vi "FE FF Frame Decoder.vi"(4 "Limit Enable(T)":bool=TRUE, 5 "INFO":T1, 6 "Test Mode":u32, 7 "Raw_Data?":bool=TRUE, 8 "error in (no error)":errorcluster, 10 "Frame Data":u8[](array[numeric]), 11 "Frame Detail":string[][](array[string])) -> (0 "error out":errorcluster, 2 "Raw Data":u64[](array[numeric]), 3 "Frame Detail With Value":string[](array[string]))   [LabVIEW 2023, in "HardwareAbstractionLayer_LVOOP.lvlib" / "Report.lvclass"]
uses:
  Report.lvclass
  Control/FE FF DECODER.ctl
  Control/ERROR LOG.ctl
  Control/TEST RESULT LOG.ctl
  Control/All Log Details.ctl
  Control/UUT Test Info.ctl
  Control/FE FRAME LOG.ctl
  Control/FF FRAME LOG.ctl
  Control/LIMIT TABLE.ctl
  Control/ERROR LOG APPEND.ctl
  Control/FA FRAME LOG.ctl
  Control/TEST RESULT LOG APPEND.ctl
  Control/SYSTEM LOG.ctl
  Control/Temperature LOG.ctl
  Control/POWER STATUS.ctl
  Control/CYCLE_DURATION_LOG.ctl
  <vilib>/Utility/error.llb/Trim Whitespace One-Sided.vi
  Report.lvclass/Report.ctl
  Database/Database.lvclass
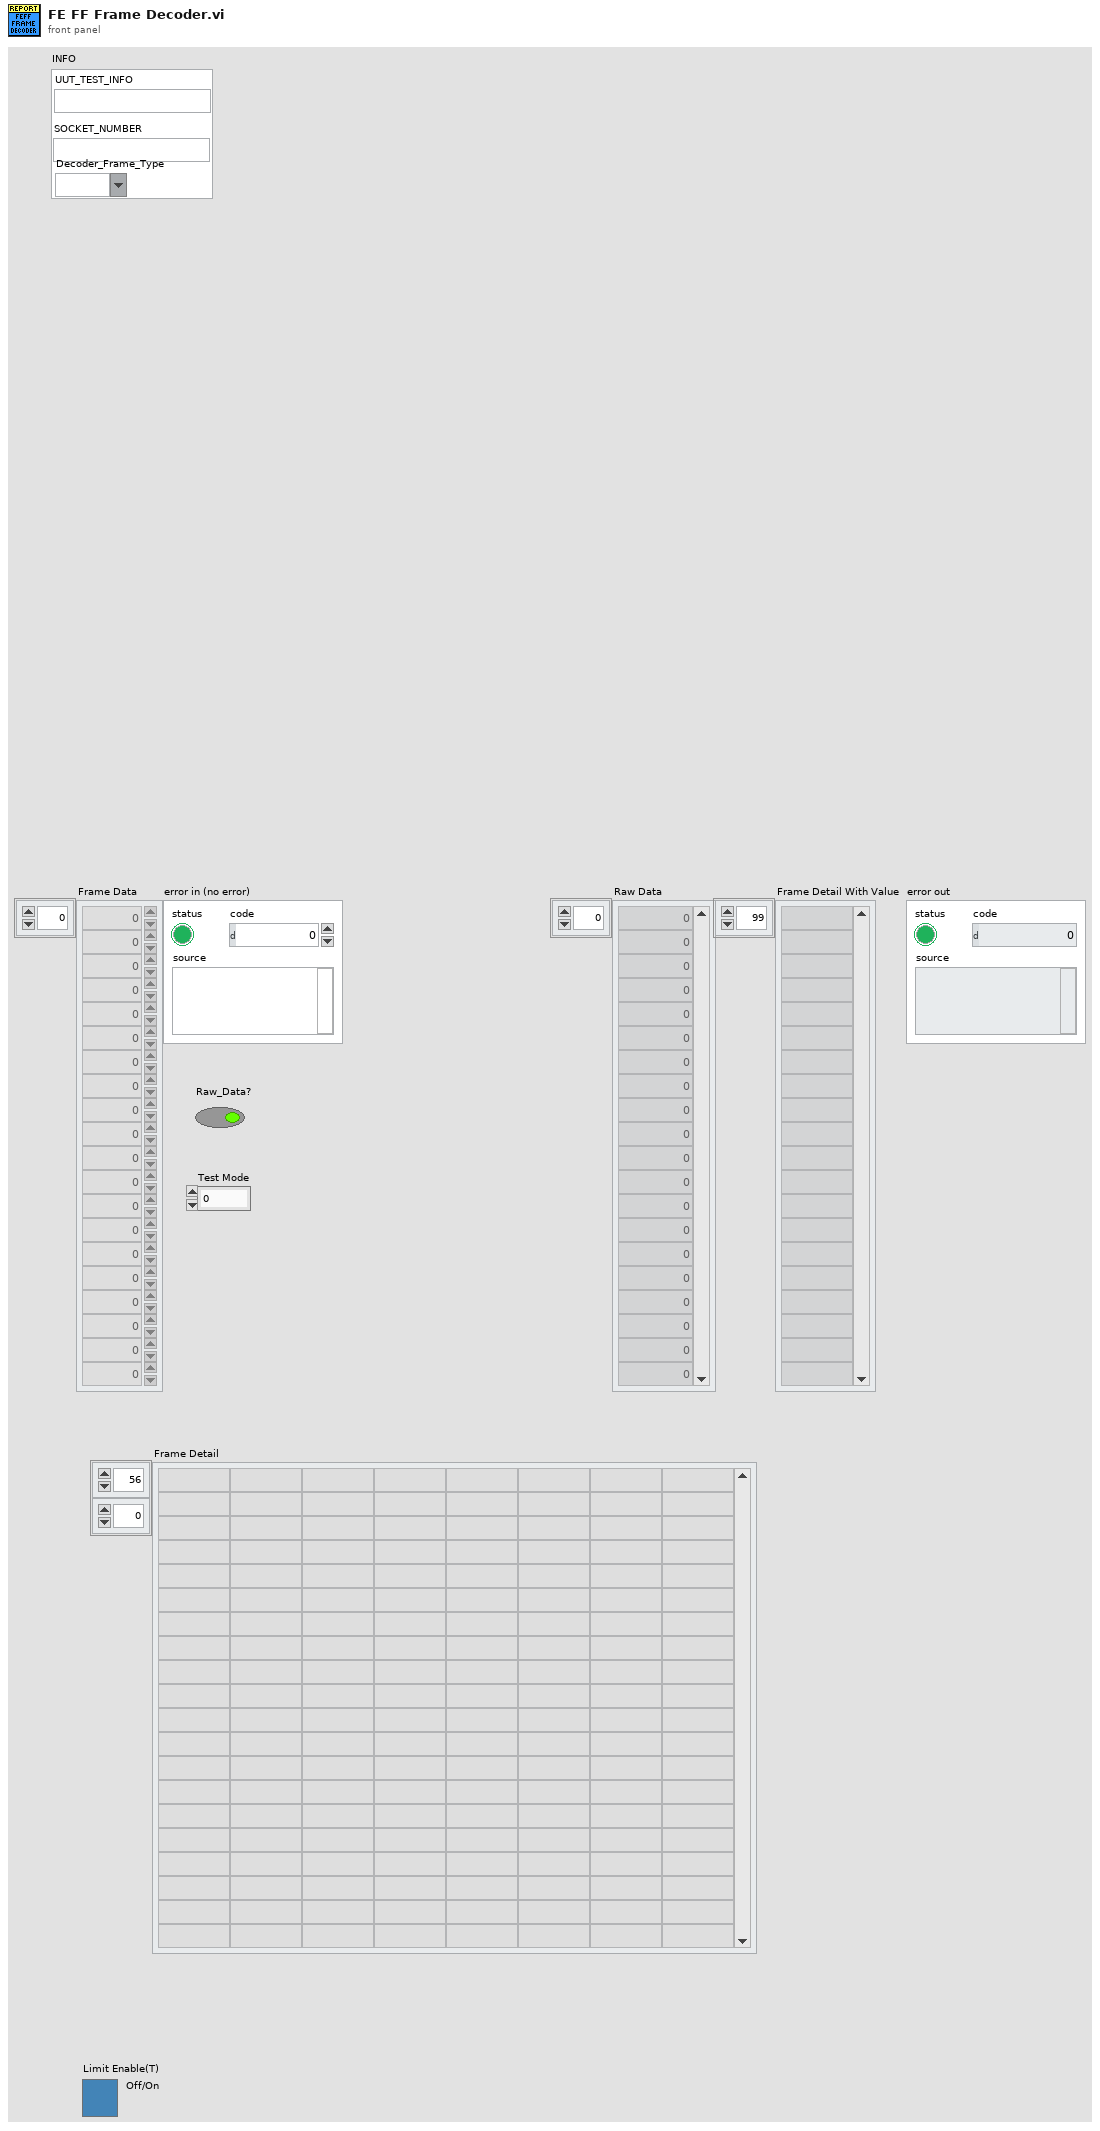
[diagram p1: front panel]
types:
  T1 = typedef "HardwareAbstractionLayer_LVOOP.lvlib/Report.lvclass/FE FF DECODER.ctl" = cluster{"UUT_TEST_INFO":string, "SOCKET_NUMBER":string, "Decoder_Frame_Type":string}
  T2 = typedef "HardwareAbstractionLayer_LVOOP.lvlib/Report.lvclass/TEST RESULT LOG.ctl" = cluster{"ID":string, "UUT_TEST_INFO":string, "DATE_TIME":string, "CYCLE_NUMBER":string, "TEST_MODE":string, "SIGNAL_NAME":string, "SIGNAL_VALUE":string, "COMPARISON_VALUE":string, "ERROR_MESSAGE":string, "FRAME_TYPE":string, "LIMITID":string, "TEST_RESULT":string, "SOCKET_NUMBER":string}
  T3 = typedef "HardwareAbstractionLayer_LVOOP.lvlib/Report.lvclass/ERROR LOG.ctl" = cluster{"ID":string, "UUT_TEST_INFO":string, "DATE_TIME":string, "CYCLE_NUMBER":string, "TEST_MODE":string, "SIGNAL_NAME":string, "SIGNAL_VALUE":string, "UNIT":string, "COMPARISON_VALUE":string, "ERROR_MESSAGE":string, "FRAME_TYPE":string, "LIMITID":string, "SOCKET_NUMBER":string}
  T4 = typedef "HardwareAbstractionLayer_LVOOP.lvlib/Report.lvclass/Result FGV Data.ctl" = cluster{"Project Name":string, "Product Name":string, "Product Varient":string, "Test Name":string, "Test Phase":string, "Test Description":string, "Temp Chamber Name":string, "Schema":string, "Total No of Cycles":u32, "Current Cycle Number":u32, "Cycle Duration":u32, "Current Test Mode":string}
  T5 = enum16{"big-endian, network order", "native, host order", "little-endian"}
  T6 = typedef "HardwareAbstractionLayer_LVOOP.lvlib/Report.lvclass/All Log Details.ctl" = cluster{"UUT_TEST_INFO":T7, "FE_FRAME_LOG":T8, "FF_FRAME_LOG":T9, "LIMIT_TABLE":T10, "ERROR LOG Append":T11, "FA_FRAME_LOG":T12, "Socket No":u16, "TEST RESULT LOG Append":T13, "SYSTEM_LOG":T14, "Temperature log":T15, "POWER_STATUS":T16, "CYCLE_DURATION_LOG":T17}
  T7 = typedef "HardwareAbstractionLayer_LVOOP.lvlib/Report.lvclass/UUT Test Info.ctl" = cluster{"ID":string, "STATION_ID":string, "TEST_SOCKET_INDEX":string, "UUT_SERIAL_NUMBER":string, "TSW_VER":string, "VAL_SW_VER":string, "PROJECT_NAME":string, "PRODUCT_NAME":string, "PRODUCT_VARIANT":string, "TEST_NAME":string, "TEST_PHASE":string, "TEST_DESCRIPTION":string, "TEMP_CHAMBER_NAME":string, "START_DATE_TIME":string, "STOP_DATE_TIME ":string, "START_CYCLE_COUNT":string, "STOP_CYCLE_COUNT":string, "EXECUTION_TIME":string, "UUT_STATUS":string, "UUT_ERROR_CODE":string, "UUT_ERROR_MESSAGE":string, "TEST_SEQUENCE":string}
  T8 = typedef "HardwareAbstractionLayer_LVOOP.lvlib/Report.lvclass/FE FRAME LOG.ctl" = cluster{"ID":string, "UUT_TEST_INFO":string, "DATE_TIME":string, "CYCLE_NUMBER":string, "TEST_MODE":string, "CHAMBER_TEMP":string, "CAN_FRAME_RX":string, "Test Mode":u32, "LV_PPS_VOLTAGE":string, "LV_PPS_CURRENT":string, "HV_PPS_VOLTAGE":string, "HV_PPS_CURRENT":string, "SOCKET_NUMBER":string, "CAN_FRAME_RX_NO_OFF_BYTE":string}
  T9 = typedef "HardwareAbstractionLayer_LVOOP.lvlib/Report.lvclass/FF FRAME LOG.ctl" = cluster{"ID":string, "UUT_TEST_INFO":string, "DATE_TIME":string, "CYCLE_NUMBER":string, "TEST_MODE":string, "CAN_FRAME_RX":string, "CHAMBER_TEMP":string, "TestMode":u32, "SOCKET_NUMBER":string, "CAN_FRAME_RX_NO_OFF_BYTE":string}
  T10 = typedef "HardwareAbstractionLayer_LVOOP.lvlib/Report.lvclass/LIMIT TABLE.ctl" = cluster{"ID":string, "PRODUCT_NAME":string, "PRODUCT_VARIANT":string, "TEST_MODE":string, "PARAMETER_NAME":string, "COMPARISON_TYPE":string, "LOW_LIMIT":string, "HIGH_LIMIT":string, "UNIT":string, "ERROR_MESSSAGE":string, "SEVERITY":string}
  T11 = typedef "HardwareAbstractionLayer_LVOOP.lvlib/Report.lvclass/ERROR LOG APPEND.ctl" = T3[]
  T12 = typedef "HardwareAbstractionLayer_LVOOP.lvlib/Report.lvclass/FA FRAME LOG.ctl" = cluster{"UUT_TEST_INFO":string, "CAN_FRAME_RX":string, "CAN_FRAME_RX_NO_OFF_BYTE":string}
  T13 = typedef "HardwareAbstractionLayer_LVOOP.lvlib/Report.lvclass/TEST RESULT LOG APPEND.ctl" = T2[]
  T14 = typedef "HardwareAbstractionLayer_LVOOP.lvlib/Report.lvclass/SYSTEM LOG.ctl" = cluster{"ID ":string, "DATE_TIME":string, "CYCLE_NUMBER":string, "TEST_MODE":string, "ERROR_MESSAGE":string}
  T15 = typedef "HardwareAbstractionLayer_LVOOP.lvlib/Report.lvclass/Temperature LOG.ctl" = cluster{"TEST_MODE":string, "CYCLE_NUMBER":string, "TEMPERATURE":cluster{"LV_PPS_TEMPERATURE":dbl, "HV_PPS1_TEMPERATURE":dbl, "HV_PPS2_TEMPERATURE":dbl, "HV_PPS3_TEMPERATURE":dbl, "HV_PPS4_TEMPERATURE":dbl, "HV_PPS5_TEMPERATURE":dbl, "HV_PPS6_TEMPERATURE":dbl, "CHAMBER_TEMPERATURE":dbl, "LOAD_U1_TEMPERATURE":dbl, "LOAD_V1_TEMPERATURE":dbl, "LOAD_W1_TEMPERATURE":dbl, "LOAD_U2_TEMPERATURE":dbl, "LOAD_V2_TEMPERATURE":dbl, "LOAD_W2_TEMPERATURE":dbl, "LOAD_U3_TEMPERATURE":dbl, "LOAD_V3_TEMPERATURE":dbl, "LOAD_W3_TEMPERATURE":dbl}, "Temperature Inrange":cluster{"LVPPS_Trip?":bool, "HVPPS1_Trip?":bool, "HVPPS2_Trip?":bool, "HVPPS3_Trip?":bool, "HVPPS4_Trip?":bool, "HVPPS5_Trip?":bool, "HVPPS6_Trip?":bool, "Chamber_Trip?":bool}}
  T16 = typedef "HardwareAbstractionLayer_LVOOP.lvlib/Report.lvclass/POWER STATUS.ctl" = cluster{"TEST_MODE":string, "CYCLE_NUMBER":string, "TYPE_POWER":string, "STATE":string}
  T17 = typedef "HardwareAbstractionLayer_LVOOP.lvlib/Report.lvclass/CYCLE_DURATION_LOG.ctl" = cluster{"CYCLE_NUMBER":string}
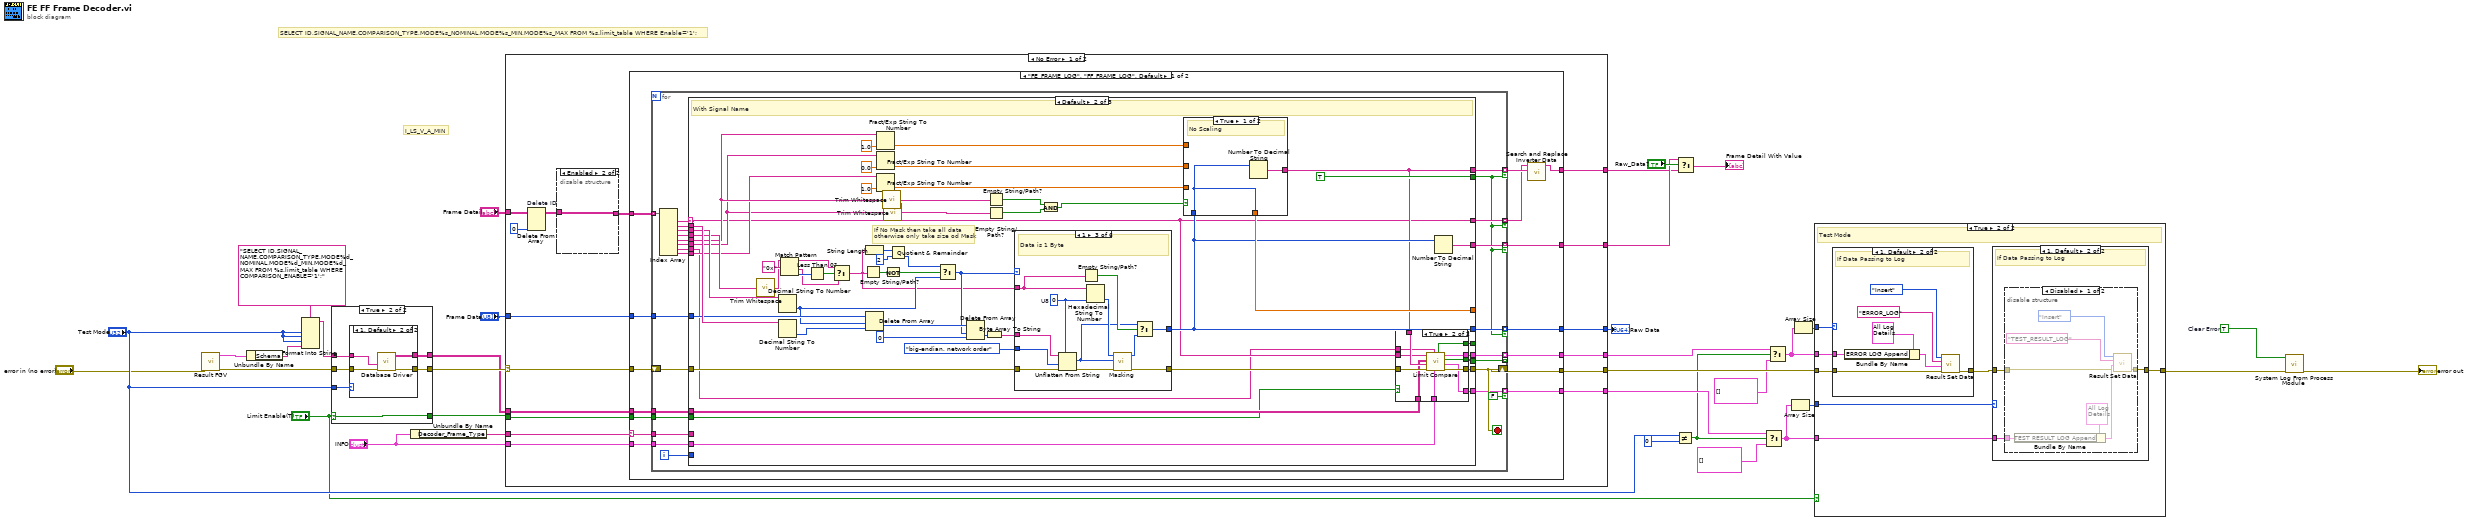
[diagram p0: block diagram]
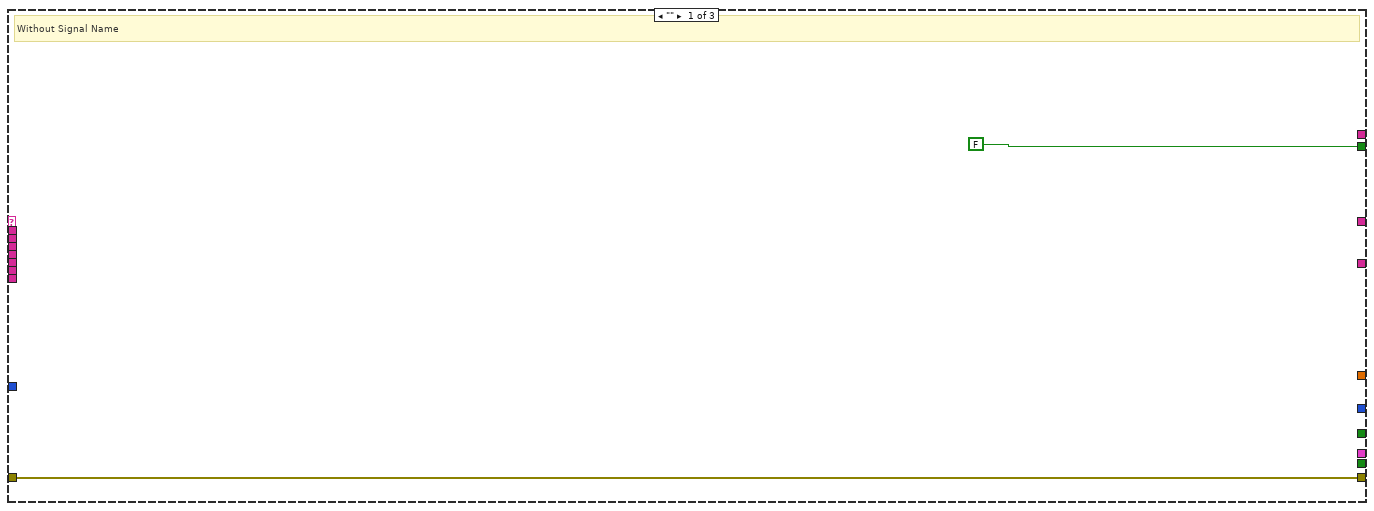
[diagram p8: hidden frame]
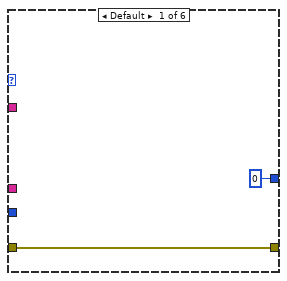
[diagram p10: hidden frame]
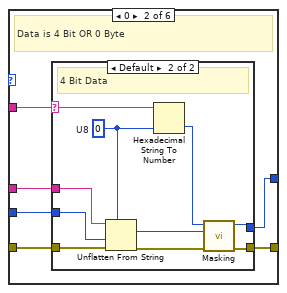
[diagram p11: hidden frame]
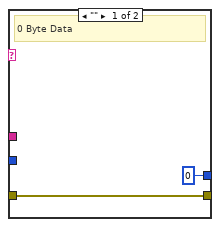
[diagram p12: hidden frame]
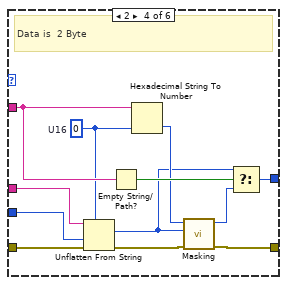
[diagram p13: hidden frame]
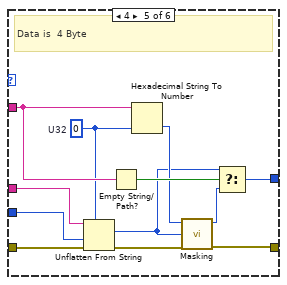
[diagram p14: hidden frame]
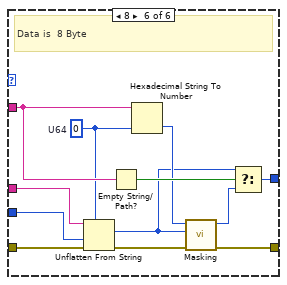
[diagram p15: hidden frame]
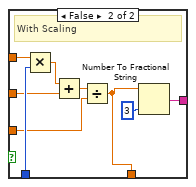
[diagram p16: hidden frame]
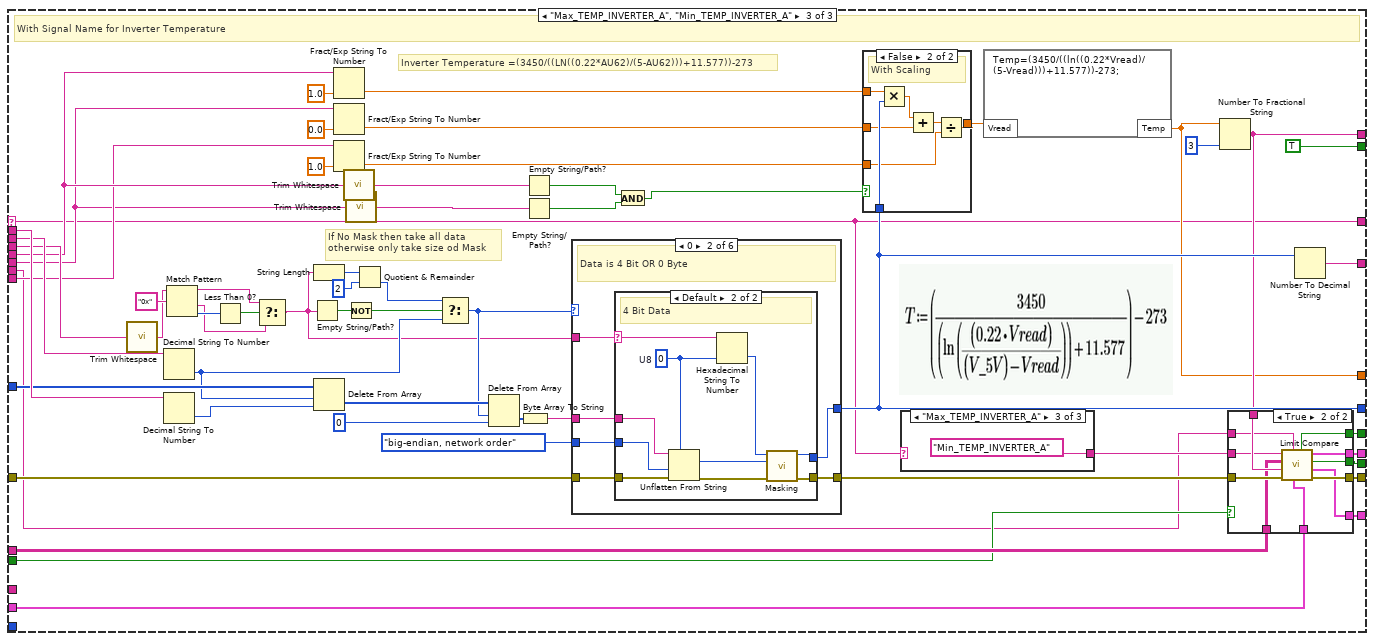
[diagram p17: hidden frame]
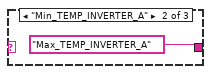
[diagram p19: hidden frame]
diagram:
  w1 = TRUE  # Clear Error
  # "I_LS_V_A_MIN"
  # "SELECT ID,SIGNAL_NAME,COMPARISON_TYPE,MODE%s_NOMINAL,MODE%s_MIN,MODE%s_MAX FROM %s.limit_table WHERE Enable='1';"
  n1 = call "Result FGV.vi"("error in"="error in (no error)") -> ("error out"=w25:errorcluster, "Result FGV Data Out"=w24:T4)  [unwired: 9 in]
  n2 = Unbundle By Name(w24) -> ("Schema"=w23:string)
  n3 = Format Into String(format string="SELECT ID,SIGNAL_NAME,COMPARISON_TYPE,MODE%d_NOMINAL,MODE%d_MIN,MODE%d_MAX FROM %s.limit_table WHERE COMPARISON_ENABLE='1';", "Test Mode", "Test Mode", "Test Mode", w23) -> (resulting string=w26:string)  [unwired: 2 in, 1 out]
  n4 = case shown="True" "Limit Enable(T)" {
    selector: "Limit Enable(T)" -> [w35 w37]
    tunnel: [w36 w42] -> w28
    tunnel: w26 -> [_ w41]
    tunnel: w25 -> [w36 w40]
    tunnel: [_ w39] -> w22
    tunnel: "Test Mode" -> [_ w38]
    tunnel: [w35 w37] -> w16
    frame False {
    }
    frame True {
      n5 = case shown="1, Default" w38 {
        tunnel: [w43 w47] -> w42
        tunnel: w41 -> [_ w46]
        tunnel: w40 -> [w43 w45]
        tunnel: [_ w44] -> w39
        frame 0 {
        }
        frame 1, Default {
          n6 = call "Database Driver.vi"("error in"=w45, "SQL query"=w46) -> ("error out"=w47:errorcluster, "data"=w44:string[][])  [unwired: 6 in, 2 out]
        }
      }
    }
  }
  n7 = Unbundle By Name("INFO") -> ("Decoder_Frame_Type"=w11:string)
  n8 = case shown="No Error" w28 {
    selector: w28 -> [w55 w443]
    tunnel: "Frame Detail" -> [w63 _]
    tunnel: [w59 w443] -> w21
    tunnel: [w58 w441] -> w29
    tunnel: "Frame Data" -> [w57 _]
    tunnel: [w56 u8[] [] ("ResponseData")] -> w34
    tunnel: [w54 w441] -> w30
    tunnel: w11 -> [w53 _]
    tunnel: w22 -> [w52 _]
    tunnel: [w51 _] -> w19
    tunnel: w16 -> [w50 _]
    tunnel: [w49 _] -> w14
    tunnel: "INFO" -> [w48 _]
    frame No Error {
      n9 = Delete From Array "Delete ID"(array=w63, index (col)=0 ("disabled index (col)")) -> (array with subset deleted=w61:string[][])  [unwired: 2 in, 1 out]
      n10 = disable-structure shown="Enabled" {
        disable-tunnel: [w439 w440] -> w62
        disable-tunnel: w61 -> [w437 w440]
        frame Disabled {
          n11 = Delete From Array "Delete Header"(array=w437, index (row)=0) -> (array with subset deleted=w439:string[][])  [unwired: 2 in, 1 out]
        }
        frame Enabled {
        }
      }
      n12 = case shown="\"FE_FRAME_LOG\", \"FF_FRAME_LOG\", Default" w53 {
        selector: w53 -> [w71 _]
        tunnel: w62 -> [w78 w409]
        tunnel: [w77 w408] -> w59
        tunnel: [w64 w407] -> w58
        tunnel: w57 -> [w76 w406]
        tunnel: [w75 u64[] []] -> w56
        tunnel: w55 -> [w74 w405]
        tunnel: [w66 w404] -> w54
        tunnel: w52 -> [w73 _]
        tunnel: [w72 T3[] []] -> w51
        tunnel: w50 -> [w70 _]
        tunnel: [w69 _] -> w49
        tunnel: w48 -> [w68 _]
        frame "FE_FRAME_LOG", "FF_FRAME_LOG", Default {
          n13 = for {
            tunnel: w78 -> [w104] mode=indexing
            tunnel: w76 -> [w101]
            shift-right: [w96] -> w77
            shift-left: w74 -> [w97]
            tunnel: [w95] -> w67 mode=indexing if=w80
            tunnel: [w94] -> w75 mode=indexing if=w80
            tunnel: [w93] -> w66 mode=indexing if=w80
            tunnel: w73 -> [w89]
            tunnel: [w85] -> w72 mode=indexing if=w88
            tunnel: [w88] -> _ mode=indexing
            tunnel: w71 -> [w87]
            tunnel: w70 -> [w86]
            tunnel: [w84] -> w69 mode=indexing if=FALSE
            tunnel: w68 -> [w83]
            tunnel: [w81] -> w65 mode=indexing if=w80
            i -> [w82]
            stop <- w96 stop-if-true
            n14 = Index Array(array=w104) -> (element #1=w92:string, element #2=w103:string, element #3=w102:string, element #4=w100:string, element #5=w98:string, element #6=w99:string, element #7=w91:string, element #8=w90:string)  [unwired: 8 in]
            n15 = case shown="Default" w92 {
              selector: w92 -> [_ w108 w254]
              tunnel: w103 -> [_ w161 w310]
              tunnel: w102 -> [_ w160 w309]
              tunnel: w101 -> [_ w159 w308]
              tunnel: w100 -> [_ w157 w306]
              tunnel: w99 -> [_ w114 w265]
              tunnel: w98 -> [_ w153 w302]
              tunnel: w97 -> [w106 w150 w299]
              tunnel: [w106 w123 w273] -> w96
              tunnel: [_ w122 w259] -> w95
              tunnel: [_ w140 w257] -> _
              tunnel: [_ w139 w289] -> w94
              tunnel: [_ w138 w288] -> w93
              tunnel: [FALSE TRUE TRUE] -> w80
              tunnel: w91 -> [_ w107 w253]
              tunnel: w90 -> [_ w129 w279]
              tunnel: w89 -> [_ w121 w272]
              tunnel: [_ w120 w271] -> w85
              tunnel: [_ w119 w270] -> w88
              tunnel: w87 -> [_ _ _]
              tunnel: w86 -> [_ w118 w269]
              tunnel: [_ w117 w268] -> w84
              tunnel: [_ w116 w267] -> _
              tunnel: w83 -> [_ w109 w256]
              tunnel: w82 -> [_ _ _]
              tunnel: [_ w108 w254] -> w81
              frame "" {
                # "Without Signal Name"
              }
              frame Default {
                # "If No Mask then take all data\notherwise only take size od Mask"
                # "With Signal Name"
                n16 = call <vilib>:"Trim Whitespace.vi"("string"=w157) -> ("trimmed string"=w136:string)  [unwired: 1 in]
                n17 = Decimal String To Number(string=w160) -> (number=w144:i32)  [unwired: 2 in, 1 out]
                n18 = Decimal String To Number(string=w161) -> (number=w158:i32)  [unwired: 2 in, 1 out]
                n19 = Match Pattern(string=w136, regular expression="0x") -> (before substring=w133:string, after substring=w132:string, offset past match=w134:i32)  [unwired: 1 in, 1 out]
                n20 = Less Than 0?(x=w134) -> (x < 0?=w135:bool)
                n21 = Select(t=w133, s=w135, f=w132) -> (s? t:f=w131:string)
                n22 = Empty String/Path?(string/path=w131) -> (empty?=w146:bool)
                n23 = String Length(string=w131) -> (length=w152:i32)
                n24 = Delete From Array(array=w159, length=w144, index=w158) -> (deleted portion=w156:u8[])  [unwired: 1 out]
                n25 = Fract/Exp String To Number(string=w153, default (0 dbl)=1.0 ("default (0 DBL)")) -> (number=w155:dbl)  [unwired: 2 in, 1 out]
                n26 = Fract/Exp String To Number(string=w114, default (0 dbl)=0.0 ("default (0 DBL)")) -> (number=w154:dbl)  [unwired: 2 in, 1 out]
                n27 = Fract/Exp String To Number(string=w129, default (0 dbl)=1.0 ("default (0 DBL)")) -> (number=w125:dbl)  [unwired: 2 in, 1 out]
                n28 = call <vilib>:"Trim Whitespace.vi"("string"=w153) -> ("trimmed string"=w115:string)  [unwired: 1 in]
                n29 = call <vilib>:"Trim Whitespace.vi"("string"=w114) -> ("trimmed string"=w113:string)  [unwired: 1 in]
                n30 = Not(x=w146) -> (.not. x?=w143:bool)
                n31 = Quotient & Remainder(x=w152, y=2) -> (floor(x/y)=w145:i32)  [unwired: 1 out]
                n32 = Select(t=w145, s=w143, f=w144) -> (s? t:f=w141:i32)
                n33 = Delete From Array(array=w156, length=w141, index=0) -> (deleted portion=w148:u8[])  [unwired: 1 out]
                n34 = Byte Array To String(unsigned byte array=w148) -> (string=w142:string)
                n35 = Empty String/Path?(string/path=w115) -> (empty?=w112:bool)
                n36 = Empty String/Path?(string/path=w113) -> (empty?=w111:bool)
                n37 = case shown="1" w141 {
                  tunnel: T5."big-endian, network order" ("byte order (0:big-endian, network order)") -> [_ w181 w205 w217 w229 w241]
                  tunnel: w150 -> [w175 w180 w204 w216 w228 w240]
                  tunnel: [w175 w179 w195 w207 w219 w230] -> w124
                  tunnel: w131 -> [_ w178 w203 w215 w227 w239]
                  tunnel: [u8 0 ("U8") w176 w201 w213 w225 w237] -> w139
                  tunnel: w142 -> [_ w177 w200 w212 w224 w236]
                  frame Default {
                  }
                  frame 0 {
                    # "Data is 4 Bit OR 0 Byte"
                    n38 = case shown="Default" w178 {
                      selector: w178 -> [_ w191]
                      tunnel: w181 -> [_ w193]
                      tunnel: w180 -> [w182 w192]
                      tunnel: [w182 w184] -> w179
                      tunnel: w177 -> [_ w190]
                      tunnel: [u8 0 w186] -> w176
                      frame "" {
                        # "0 Byte Data"
                      }
                      frame Default {
                        w189 = u8 0  # U8
                        # "4 Bit Data"
                        n39 = Unflatten From String(type=w189, binary string=w190, byte order (0:big-endian, network order)=w193, error in (no error)=w192) -> (value=w187:u8, error out=w185:errorcluster)  [unwired: 1 in, 1 out]
                        n40 = Hexadecimal String To Number(string=w191, default (0uL)=w189) -> (number=w188:u8)  [unwired: 1 in, 1 out]
                        n41 = call "Masking.vi"("error in"=w185, "Number"=w187, "Mask in"=w188) -> ("error out"=w184:errorcluster, "Mask Data"=w186:u32)  [unwired: 6 in, 1 out]
                      }
                    }
                  }
                  frame 1 {
                    w199 = u8 0  # U8
                    # "Data is 1 Byte"
                    n42 = Unflatten From String(type=w199, binary string=w200, byte order (0:big-endian, network order)=w205, error in (no error)=w204) -> (value=w197:u8, error out=w196:errorcluster)  [unwired: 1 in, 1 out]
                    n43 = Empty String/Path?(string/path=w203) -> (empty?=w202:bool)
                    n44 = Hexadecimal String To Number(string=w203, default (0uL)=w199) -> (number=w198:u8)  [unwired: 1 in, 1 out]
                    n45 = call "Masking.vi"("error in"=w196, "Number"=w197, "Mask in"=w198) -> ("error out"=w195:errorcluster, "Mask Data"=w194:u32)  [unwired: 6 in, 1 out]
                    n46 = Select(t=w197, s=w202, f=w194) -> (s? t:f=w201:u32)
                  }
                  frame 2 {
                    w211 = u16 0  # U16
                    # "Data is  2 Byte"
                    n47 = Unflatten From String(type=w211, binary string=w212, byte order (0:big-endian, network order)=w217, error in (no error)=w216) -> (value=w209:u16, error out=w208:errorcluster)  [unwired: 1 in, 1 out]
                    n48 = Empty String/Path?(string/path=w215) -> (empty?=w214:bool)
                    n49 = Hexadecimal String To Number(string=w215, default (0uL)=w211) -> (number=w210:u16)  [unwired: 1 in, 1 out]
                    n50 = call "Masking.vi"("error in"=w208, "Number"=w209, "Mask in"=w210) -> ("error out"=w207:errorcluster, "Mask Data"=w206:u32)  [unwired: 6 in, 1 out]
                    n51 = Select(t=w209, s=w214, f=w206) -> (s? t:f=w213:u32)
                  }
                  frame 4 {
                    w223 = u32 0  # U32
                    # "Data is  4 Byte"
                    n52 = Unflatten From String(type=w223, binary string=w224, byte order (0:big-endian, network order)=w229, error in (no error)=w228) -> (value=w221:u32, error out=w220:errorcluster)  [unwired: 1 in, 1 out]
                    n53 = Empty String/Path?(string/path=w227) -> (empty?=w226:bool)
                    n54 = Hexadecimal String To Number(string=w227, default (0uL)=w223) -> (number=w222:u32)  [unwired: 1 in, 1 out]
                    n55 = call "Masking.vi"("error in"=w220, "Number"=w221, "Mask in"=w222) -> ("error out"=w219:errorcluster, "Mask Data"=w218:u32)  [unwired: 6 in, 1 out]
                    n56 = Select(t=w221, s=w226, f=w218) -> (s? t:f=w225:u32)
                  }
                  frame 8 {
                    w235 = u64 0  # U64
                    # "Data is  8 Byte"
                    n57 = Unflatten From String(type=w235, binary string=w236, byte order (0:big-endian, network order)=w241, error in (no error)=w240) -> (value=w233:u64, error out=w232:errorcluster)  [unwired: 1 in, 1 out]
                    n58 = Empty String/Path?(string/path=w239) -> (empty?=w238:bool)
                    n59 = Hexadecimal String To Number(string=w239, default (0uL)=w235) -> (number=w234:u64)  [unwired: 1 in, 1 out]
                    n60 = call "Masking.vi"("error in"=w232, "Number"=w233, "Mask in"=w234) -> ("error out"=w230:errorcluster, "Mask Data"=w231:u32)  [unwired: 6 in, 1 out]
                    n61 = Select(t=w233, s=w238, f=w231) -> (s? t:f=w237:u64)
                  }
                }
                n62 = And(x=w112, y=w111) -> (x .and. y?=w110:bool)
                n63 = case shown="True" w110 {
                  tunnel: w139 -> [w242 w251]
                  tunnel: w155 -> [_ w250]
                  tunnel: w154 -> [_ w249]
                  tunnel: [w243 w248] -> w122
                  tunnel: [w242 w245] -> w140
                  tunnel: w125 -> [_ w244]
                  frame True {
                    # "No Scaling"
                    n64 = Number To Decimal String(number=w242) -> (decimal integer string=w243:string)  [unwired: 1 in]
                  }
                  frame False {
                    # "With Scaling"
                    n65 = Multiply(x=w250, y=w251) -> (x*y=w252:dbl)
                    n66 = Add(x=w252, y=w249) -> (x+y=w246:dbl)
                    n67 = Divide(x=w246, y=w244) -> (x/y=w245:dbl)
                    n68 = Number To Fractional String(number=w245, precision (6)=i16 3) -> (F-format string=w248:string)  [unwired: 2 in]
                  }
                }
                n69 = case shown="True" w118 {
                  tunnel: w124 -> [w162 w173]
                  tunnel: [w162 w172] -> w123
                  tunnel: w122 -> [_ w171]
                  tunnel: w108 -> [_ w170]
                  tunnel: w121 -> [_ w169]
                  tunnel: [_ w168] -> w120
                  tunnel: [_ w167] -> w119
                  tunnel: [_ w166] -> w117
                  tunnel: [_ w165] -> w116
                  tunnel: w109 -> [_ w164]
                  tunnel: w107 -> [_ w163]
                  frame False {
                  }
                  frame True {
                    n70 = call "Limit Compare.vi"("INFO"=w164, "Unit"=w163, "error in"=w173, "Input Data"=w171, "Limit Signal"=w169, "Signal Name"=w170) -> ("error out"=w172:errorcluster, "TEST RESULT LOG"=w166:T2, "Out range?"=w167:bool, "ERROR_LOG"=w168:T3, "Log?"=w165:bool)  [unwired: 1 in]
                  }
                }
                n71 = Number To Decimal String(number=w139) -> (decimal integer string=w138:string)  [unwired: 1 in]
              }
              frame "Max_TEMP_INVERTER_A", "Min_TEMP_INVERTER_A" {
                # "Formual Temp"
                # "Inverter Temperature =(3450/((LN((0.22*AU62)/(5-AU62)))+11.577))-273"
                # "If No Mask then take all data\notherwise only take size od Mask"
                # "With Signal Name for Inverter Temperature"
                n72 = call <vilib>:"Trim Whitespace.vi"("string"=w306) -> ("trimmed string"=w286:string)  [unwired: 1 in]
                n73 = Decimal String To Number(string=w309) -> (number=w293:i32)  [unwired: 2 in, 1 out]
                n74 = Decimal String To Number(string=w310) -> (number=w307:i32)  [unwired: 2 in, 1 out]
                n75 = Match Pattern(string=w286, regular expression="0x") -> (before substring=w283:string, after substring=w282:string, offset past match=w284:i32)  [unwired: 1 in, 1 out]
                n76 = Less Than 0?(x=w284) -> (x < 0?=w285:bool)
                n77 = Select(t=w283, s=w285, f=w282) -> (s? t:f=w281:string)
                n78 = Empty String/Path?(string/path=w281) -> (empty?=w295:bool)
                n79 = String Length(string=w281) -> (length=w301:i32)
                n80 = Delete From Array(array=w308, length=w293, index=w307) -> (deleted portion=w305:u8[])  [unwired: 1 out]
                n81 = Fract/Exp String To Number(string=w302, default (0 dbl)=1.0 ("default (0 DBL)")) -> (number=w304:dbl)  [unwired: 2 in, 1 out]
                n82 = Fract/Exp String To Number(string=w265, default (0 dbl)=0.0 ("default (0 DBL)")) -> (number=w303:dbl)  [unwired: 2 in, 1 out]
                n83 = Fract/Exp String To Number(string=w279, default (0 dbl)=1.0 ("default (0 DBL)")) -> (number=w275:dbl)  [unwired: 2 in, 1 out]
                n84 = call <vilib>:"Trim Whitespace.vi"("string"=w302) -> ("trimmed string"=w266:string)  [unwired: 1 in]
                n85 = call <vilib>:"Trim Whitespace.vi"("string"=w265) -> ("trimmed string"=w264:string)  [unwired: 1 in]
                n86 = Not(x=w295) -> (.not. x?=w292:bool)
                n87 = Quotient & Remainder(x=w301, y=2) -> (floor(x/y)=w294:i32)  [unwired: 1 out]
                n88 = Select(t=w294, s=w292, f=w293) -> (s? t:f=w290:i32)
                n89 = Delete From Array(array=w305, length=w290, index=0) -> (deleted portion=w297:u8[])  [unwired: 1 out]
                n90 = Byte Array To String(unsigned byte array=w297) -> (string=w291:string)
                n91 = Empty String/Path?(string/path=w266) -> (empty?=w263:bool)
                n92 = Empty String/Path?(string/path=w264) -> (empty?=w262:bool)
                n93 = case shown="0" w290 {
                  tunnel: T5."big-endian, network order" ("byte order (0:big-endian, network order)") -> [_ w333 w357 w369 w381 w393]
                  tunnel: w299 -> [w327 w332 w356 w368 w380 w392]
                  tunnel: [w327 w331 w347 w359 w371 w382] -> w274
                  tunnel: w281 -> [_ w330 w355 w367 w379 w391]
                  tunnel: [u8 0 ("U8") w328 w353 w365 w377 w389] -> w289
                  tunnel: w291 -> [_ w329 w352 w364 w376 w388]
                  frame Default {
                  }
                  frame 0 {
                    # "Data is 4 Bit OR 0 Byte"
                    n94 = case shown="Default" w330 {
                      selector: w330 -> [_ w343]
                      tunnel: w333 -> [_ w345]
                      tunnel: w332 -> [w334 w344]
                      tunnel: [w334 w336] -> w331
                      tunnel: w329 -> [_ w342]
                      tunnel: [u8 0 w338] -> w328
                      frame "" {
                        # "0 Byte Data"
                      }
                      frame Default {
                        w341 = u8 0  # U8
                        # "4 Bit Data"
                        n95 = Unflatten From String(type=w341, binary string=w342, byte order (0:big-endian, network order)=w345, error in (no error)=w344) -> (value=w339:u8, error out=w337:errorcluster)  [unwired: 1 in, 1 out]
                        n96 = Hexadecimal String To Number(string=w343, default (0uL)=w341) -> (number=w340:u8)  [unwired: 1 in, 1 out]
                        n97 = call "Masking.vi"("error in"=w337, "Number"=w339, "Mask in"=w340) -> ("error out"=w336:errorcluster, "Mask Data"=w338:u32)  [unwired: 6 in, 1 out]
                      }
                    }
                  }
                  frame 1 {
                    w351 = u8 0  # U8
                    # "Data is 1 Byte"
                    n98 = Unflatten From String(type=w351, binary string=w352, byte order (0:big-endian, network order)=w357, error in (no error)=w356) -> (value=w349:u8, error out=w348:errorcluster)  [unwired: 1 in, 1 out]
                    n99 = Empty String/Path?(string/path=w355) -> (empty?=w354:bool)
                    n100 = Hexadecimal String To Number(string=w355, default (0uL)=w351) -> (number=w350:u8)  [unwired: 1 in, 1 out]
                    n101 = call "Masking.vi"("error in"=w348, "Number"=w349, "Mask in"=w350) -> ("error out"=w347:errorcluster, "Mask Data"=w346:u32)  [unwired: 6 in, 1 out]
                    n102 = Select(t=w349, s=w354, f=w346) -> (s? t:f=w353:u32)
                  }
                  frame 2 {
                    w363 = u16 0  # U16
                    # "Data is  2 Byte"
                    n103 = Unflatten From String(type=w363, binary string=w364, byte order (0:big-endian, network order)=w369, error in (no error)=w368) -> (value=w361:u16, error out=w360:errorcluster)  [unwired: 1 in, 1 out]
                    n104 = Empty String/Path?(string/path=w367) -> (empty?=w366:bool)
                    n105 = Hexadecimal String To Number(string=w367, default (0uL)=w363) -> (number=w362:u16)  [unwired: 1 in, 1 out]
                    n106 = call "Masking.vi"("error in"=w360, "Number"=w361, "Mask in"=w362) -> ("error out"=w359:errorcluster, "Mask Data"=w358:u32)  [unwired: 6 in, 1 out]
                    n107 = Select(t=w361, s=w366, f=w358) -> (s? t:f=w365:u32)
                  }
                  frame 4 {
                    w375 = u32 0  # U32
                    # "Data is  4 Byte"
                    n108 = Unflatten From String(type=w375, binary string=w376, byte order (0:big-endian, network order)=w381, error in (no error)=w380) -> (value=w373:u32, error out=w372:errorcluster)  [unwired: 1 in, 1 out]
                    n109 = Empty String/Path?(string/path=w379) -> (empty?=w378:bool)
                    n110 = Hexadecimal String To Number(string=w379, default (0uL)=w375) -> (number=w374:u32)  [unwired: 1 in, 1 out]
                    n111 = call "Masking.vi"("error in"=w372, "Number"=w373, "Mask in"=w374) -> ("error out"=w371:errorcluster, "Mask Data"=w370:u32)  [unwired: 6 in, 1 out]
                    n112 = Select(t=w373, s=w378, f=w370) -> (s? t:f=w377:u32)
                  }
                  frame 8 {
                    w387 = u64 0  # U64
                    # "Data is  8 Byte"
                    n113 = Unflatten From String(type=w387, binary string=w388, byte order (0:big-endian, network order)=w393, error in (no error)=w392) -> (value=w385:u64, error out=w384:errorcluster)  [unwired: 1 in, 1 out]
                    n114 = Empty String/Path?(string/path=w391) -> (empty?=w390:bool)
                    n115 = Hexadecimal String To Number(string=w391, default (0uL)=w387) -> (number=w386:u64)  [unwired: 1 in, 1 out]
                    n116 = call "Masking.vi"("error in"=w384, "Number"=w385, "Mask in"=w386) -> ("error out"=w382:errorcluster, "Mask Data"=w383:u32)  [unwired: 6 in, 1 out]
                    n117 = Select(t=w385, s=w390, f=w383) -> (s? t:f=w389:u64)
                  }
                }
                n118 = And(x=w263, y=w262) -> (x .and. y?=w261:bool)
                n119 = case shown="False" w261 {
                  tunnel: w289 -> [w394 w400]
                  tunnel: w304 -> [_ w399]
                  tunnel: w303 -> [_ w398]
                  tunnel: w275 -> [_ w396]
                  tunnel: [w394 w395] -> w258
                  frame True {
                    # "No Scaling"
                  }
                  frame False {
                    # "With Scaling"
                    n120 = Multiply(x=w399, y=w400) -> (x*y=w401:dbl)
                    n121 = Add(x=w401, y=w398) -> (x+y=w397:dbl)
                    n122 = Divide(x=w397, y=w396) -> (x/y=w395:dbl)
                  }
                }
                n123 = case shown="\"Max_TEMP_INVERTER_A\"" w254 {
                  selector: w254 -> [w311 _ _]
                  tunnel: [w311 "Max_TEMP_INVERTER_A" "Min_TEMP_INVERTER_A"] -> w255
                  frame "", Default {
                  }
                  frame "Min_TEMP_INVERTER_A" {
                  }
                  frame "Max_TEMP_INVERTER_A" {
                  }
                }
                n124 = formula code="Temp=(3450/((ln((0.22*Vread)/(5-Vread)))+11.577))-273;"("Vread"=w258) -> ("Temp"=w257:dbl)
                n125 = Number To Fractional String(number=w257, precision (6)=i16 3) -> (F-format string=w259:string)  [unwired: 2 in]
                n126 = case shown="True" w269 {
                  tunnel: w274 -> [w314 w325]
                  tunnel: [w314 w324] -> w273
                  tunnel: w259 -> [_ w323]
                  tunnel: w255 -> [_ w322]
                  tunnel: w272 -> [_ w321]
                  tunnel: [_ w320] -> w271
                  tunnel: [_ w319] -> w270
                  tunnel: [_ w318] -> w268
                  tunnel: [_ w317] -> w267
                  tunnel: w256 -> [_ w316]
                  tunnel: w253 -> [_ w315]
                  frame False {
                  }
                  frame True {
                    n127 = call "Limit Compare.vi"("INFO"=w316, "Unit"=w315, "error in"=w325, "Input Data"=w323, "Limit Signal"=w321, "Signal Name"=w322) -> ("error out"=w324:errorcluster, "TEST RESULT LOG"=w318:T2, "Out range?"=w319:bool, "ERROR_LOG"=w320:T3, "Log?"=w317:bool)  [unwired: 1 in]
                  }
                }
                n128 = Number To Decimal String(number=w289) -> (decimal integer string=w288:string)  [unwired: 1 in]
              }
            }
          }
          n129 = call "Search and Replace Inverter Data.vi"("Signal Value in"=w67, "Signal Name"=w65) -> ("Signal Value out"=w64:string[])  [unwired: 9 in]
        }
        frame "FA_FRAME_LOG" {
          (unwired) dbl[] []
          n130 = for {
            tunnel: w409 -> [w425] mode=indexing
            tunnel: w406 -> [w422]
            tunnel: [w418] -> _ mode=indexing
            shift-right: [w416] -> w408
            shift-left: w405 -> [w417]
            tunnel: [w415] -> w407 mode=indexing if=w412
            tunnel: [w414] -> w404 mode=indexing if=w412
            i -> [w418]
            stop <- w416 stop-if-true
            n131 = Index Array(array=w425) -> (element #1=w413:string, element #2=w424:string, element #3=w423:string, element #4=w421:string, element #5=w419:string, element #6=w420:string, element #7=w411:string, element #8=w410:string)  [unwired: 8 in]
            n132 = case shown="Default" w413 {
              tunnel: w424 -> [_ w436]
              tunnel: w423 -> [_ w435]
              tunnel: w422 -> [_ w434]
              tunnel: w421 -> [_ _]
              tunnel: w420 -> [_ _]
              tunnel: w419 -> [_ _]
              tunnel: w417 -> [w427 w432]
              tunnel: [w427 w432] -> w416
              tunnel: [_ w428] -> w415
              tunnel: [_ w428] -> w414
              tunnel: [FALSE TRUE] -> w412
              tunnel: w411 -> [_ _]
              tunnel: w410 -> [_ _]
              frame "" {
                # "Without Signal Name"
              }
              frame Default {
                # "If No Mask then take all data\notherwise only take size od Mask"
                # "With Signal Name"
                n133 = Decimal String To Number(string=w435) -> (number=w431:i32)  [unwired: 2 in, 1 out]
                n134 = Decimal String To Number(string=w436) -> (number=w433:i32)  [unwired: 2 in, 1 out]
                n135 = Delete From Array(array=w434, length=w431, index=w433) -> (deleted portion=w429:u8[])  [unwired: 1 out]
                n136 = Byte Array To String(unsigned byte array=w429) -> (string=w428:string)
              }
            }
          }
        }
      }
    }
    frame Error {
      (unwired) dbl[] []
      w441 = string[] []
    }
  }
  "Raw Data" <- w34
  n137 = Not Equal?(x="Test Mode", y=0) -> (x != y?=w6:bool)
  n138 = Select(t=w30, s="Raw_Data?", f=w29) -> (s? t:f=→"Frame Detail With Value":string[])
  n139 = Select(t=w14, s=w6, f=T2[] []) -> (s? t:f=w3:T2[])
  n140 = Select(t=w19, s=w6, f=T3[] []) -> (s? t:f=w7:T3[])
  n141 = Array Size(array=w3) -> (size(s)=w4:i32)
  n142 = Array Size(array=w7) -> (size(s)=w9:i32)
  n143 = case shown="True" "Limit Enable(T)" {
    tunnel: w21 -> [w444 w451]
    tunnel: w9 -> [_ w450]
    tunnel: [w444 w447] -> w2
    tunnel: w7 -> [_ w449]
    tunnel: w4 -> [_ w446]
    tunnel: w3 -> [_ w445]
    frame False {
      # "Manual Mode"
    }
    frame True {
      # "Test Mode"
      n144 = case shown="1, Default" w450 {
        tunnel: w451 -> [w464 w471]
        tunnel: [w464 w470] -> w448
        tunnel: w449 -> [_ w467]
        frame 0 {
          # "Emety Data"
        }
        frame 1, Default {
          # "If Data Passing to Log"
          n145 = Bundle By Name(cluster=T6 {"UUT_TEST_INFO"={"ID"="", "STATION_ID"="", "TEST_SOCKET_INDEX"="", "UUT_SERIAL_NUMBER"="", "TSW_VER"="", "VAL_SW_VER"="", "PROJECT_NAME"="", "PRODUCT_NAME"="", "PRODUCT_VARIANT"="", "TEST_NAME"="", "TEST_PHASE"="", "TEST_DESCRIPTION"="", "TEMP_CHAMBER_NAME"="", "START_DATE_TIME"="", "STOP_DATE_TIME "="", "START_CYCLE_COUNT"="", "STOP_CYCLE_COUNT"="", "EXECUTION_TIME"="", "UUT_STATUS"="", "UUT_ERROR_CODE"="", "UUT_ERROR_MESSAGE"="", "TEST_SEQUENCE"=""}, "FE_FRAME_LOG"={"ID"="", "UUT_TEST_INFO"="", "DATE_TIME"="", "CYCLE_NUMBER"="", "TEST_MODE"="", "CHAMBER_TEMP"="", "CAN_FRAME_RX"="", "Test Mode"=0, "LV_PPS_VOLTAGE"="", "LV_PPS_CURRENT"="", "HV_PPS_VOLTAGE"="", "HV_PPS_CURRENT"="", "SOCKET_NUMBER"="", "CAN_FRAME_RX_NO_OFF_BYTE"=""}, "FF_FRAME_LOG"={"ID"="", "UUT_TEST_INFO"="", "DATE_TIME"="", "CYCLE_NUMBER"="", "TEST_MODE"="", "CAN_FRAME_RX"="", "CHAMBER_TEMP"="", "TestMode"=0, "SOCKET_NUMBER"="", "CAN_FRAME_RX_NO_OFF_BYTE"=""}, "LIMIT_TABLE"={"ID"="", "PRODUCT_NAME"="", "PRODUCT_VARIANT"="", "TEST_MODE"="", "PARAMETER_NAME"="", "COMPARISON_TYPE"="", "LOW_LIMIT"="", "HIGH_LIMIT"="", "UNIT"="", "ERROR_MESSSAGE"="", "SEVERITY"=""}, "ERROR LOG Append"=[], "FA_FRAME_LOG"={"UUT_TEST_INFO"="", "CAN_FRAME_RX"="", "CAN_FRAME_RX_NO_OFF_BYTE"=""}, "Socket No"=1, "TEST RESULT LOG Append"=[], "SYSTEM_LOG"={"ID "="", "DATE_TIME"="", "CYCLE_NUMBER"="", "TEST_MODE"="", "ERROR_MESSAGE"=""}, "Temperature log"={"TEST_MODE"="", "CYCLE_NUMBER"="", "TEMPERATURE"={"LV_PPS_TEMPERATURE"=0.0, "HV_PPS1_TEMPERATURE"=0.0, "HV_PPS2_TEMPERATURE"=0.0, "HV_PPS3_TEMPERATURE"=0.0, "HV_PPS4_TEMPERATURE"=0.0, "HV_PPS5_TEMPERATURE"=0.0, "HV_PPS6_TEMPERATURE"=0.0, "CHAMBER_TEMPERATURE"=0.0, "LOAD_U1_TEMPERATURE"=0.0, "LOAD_V1_TEMPERATURE"=0.0, "LOAD_W1_TEMPERATURE"=0.0, "LOAD_U2_TEMPERATURE"=0.0, "LOAD_V2_TEMPERATURE"=0.0, "LOAD_W2_TEMPERATURE"=0.0, "LOAD_U3_TEMPERATURE"=0.0, "LOAD_V3_TEMPERATURE"=0.0, "LOAD_W3_TEMPERATURE"=0.0}, "Temperature Inrange"={"LVPPS_Trip?"=FALSE, "HVPPS1_Trip?"=FALSE, "HVPPS2_Trip?"=FALSE, "HVPPS3_Trip?"=FALSE, "HVPPS4_Trip?"=FALSE, "HVPPS5_Trip?"=FALSE, "HVPPS6_Trip?"=FALSE, "Chamber_Trip?"=FALSE}}, "POWER_STATUS"={"TEST_MODE"="", "CYCLE_NUMBER"="", "TYPE_POWER"="", "STATE"=""}, "CYCLE_DURATION_LOG"={"CYCLE_NUMBER"=""}} ("Set Data"), "ERROR LOG Append"=w467) -> (w468:T6)
          n146 = call "Result Set Data.vi"("error in"=w471, "Set Data"=w468, "Table Name"="ERROR_LOG", "Action"=enum16{"Insert", "Update"}."Insert") -> ("error out"=w470:errorcluster)  [unwired: 7 in]
        }
      }
      n147 = case shown="1, Default" w446 {
        tunnel: w448 -> [w452 w455]
        tunnel: [w452 w454] -> w447
        tunnel: w445 -> [_ w453]
        frame 0 {
        }
        frame 1, Default {
          # "If Data Passing to Log"
          n148 = disable-structure shown="Disabled" {
            disable-tunnel: w455 -> [w458 w463]
            disable-tunnel: [w457 w463] -> w454
            disable-tunnel: w453 -> [w456 _]
            frame Disabled {
              n149 = Bundle By Name(cluster=T6 {"UUT_TEST_INFO"={"ID"="", "STATION_ID"="", "TEST_SOCKET_INDEX"="", "UUT_SERIAL_NUMBER"="", "TSW_VER"="", "VAL_SW_VER"="", "PROJECT_NAME"="", "PRODUCT_NAME"="", "PRODUCT_VARIANT"="", "TEST_NAME"="", "TEST_PHASE"="", "TEST_DESCRIPTION"="", "TEMP_CHAMBER_NAME"="", "START_DATE_TIME"="", "STOP_DATE_TIME "="", "START_CYCLE_COUNT"="", "STOP_CYCLE_COUNT"="", "EXECUTION_TIME"="", "UUT_STATUS"="", "UUT_ERROR_CODE"="", "UUT_ERROR_MESSAGE"="", "TEST_SEQUENCE"=""}, "FE_FRAME_LOG"={"ID"="", "UUT_TEST_INFO"="", "DATE_TIME"="", "CYCLE_NUMBER"="", "TEST_MODE"="", "CHAMBER_TEMP"="", "CAN_FRAME_RX"="", "Test Mode"=0, "LV_PPS_VOLTAGE"="", "LV_PPS_CURRENT"="", "HV_PPS_VOLTAGE"="", "HV_PPS_CURRENT"="", "SOCKET_NUMBER"="", "CAN_FRAME_RX_NO_OFF_BYTE"=""}, "FF_FRAME_LOG"={"ID"="", "UUT_TEST_INFO"="", "DATE_TIME"="", "CYCLE_NUMBER"="", "TEST_MODE"="", "CAN_FRAME_RX"="", "CHAMBER_TEMP"="", "TestMode"=0, "SOCKET_NUMBER"="", "CAN_FRAME_RX_NO_OFF_BYTE"=""}, "LIMIT_TABLE"={"ID"="", "PRODUCT_NAME"="", "PRODUCT_VARIANT"="", "TEST_MODE"="", "PARAMETER_NAME"="", "COMPARISON_TYPE"="", "LOW_LIMIT"="", "HIGH_LIMIT"="", "UNIT"="", "ERROR_MESSSAGE"="", "SEVERITY"=""}, "ERROR LOG Append"=[], "FA_FRAME_LOG"={"UUT_TEST_INFO"="", "CAN_FRAME_RX"="", "CAN_FRAME_RX_NO_OFF_BYTE"=""}, "Socket No"=1, "TEST RESULT LOG Append"=[], "SYSTEM_LOG"={"ID "="", "DATE_TIME"="", "CYCLE_NUMBER"="", "TEST_MODE"="", "ERROR_MESSAGE"=""}, "Temperature log"={"TEST_MODE"="", "CYCLE_NUMBER"="", "TEMPERATURE"={"LV_PPS_TEMPERATURE"=0.0, "HV_PPS1_TEMPERATURE"=0.0, "HV_PPS2_TEMPERATURE"=0.0, "HV_PPS3_TEMPERATURE"=0.0, "HV_PPS4_TEMPERATURE"=0.0, "HV_PPS5_TEMPERATURE"=0.0, "HV_PPS6_TEMPERATURE"=0.0, "CHAMBER_TEMPERATURE"=0.0, "LOAD_U1_TEMPERATURE"=0.0, "LOAD_V1_TEMPERATURE"=0.0, "LOAD_W1_TEMPERATURE"=0.0, "LOAD_U2_TEMPERATURE"=0.0, "LOAD_V2_TEMPERATURE"=0.0, "LOAD_W2_TEMPERATURE"=0.0, "LOAD_U3_TEMPERATURE"=0.0, "LOAD_V3_TEMPERATURE"=0.0, "LOAD_W3_TEMPERATURE"=0.0}, "Temperature Inrange"={"LVPPS_Trip?"=FALSE, "HVPPS1_Trip?"=FALSE, "HVPPS2_Trip?"=FALSE, "HVPPS3_Trip?"=FALSE, "HVPPS4_Trip?"=FALSE, "HVPPS5_Trip?"=FALSE, "HVPPS6_Trip?"=FALSE, "Chamber_Trip?"=FALSE}}, "POWER_STATUS"={"TEST_MODE"="", "CYCLE_NUMBER"="", "TYPE_POWER"="", "STATE"=""}, "CYCLE_DURATION_LOG"={"CYCLE_NUMBER"=""}} ("Set Data"), "TEST RESULT LOG Append"=w456) -> (w460:T6)
              n150 = call "Result Set Data.vi"("error in"=w458, "Set Data"=w460, "Table Name"="TEST_RESULT_LOG", "Action"=enum16{"Insert", "Update"}."Insert") -> ("error out"=w457:errorcluster)  [unwired: 7 in]
            }
            frame Enabled {
            }
          }
        }
      }
    }
  }
  n151 = call "System Log From Process Module.vi"("error in"=w2, "Clear Error"=w1) -> ("error out"=→"error out":errorcluster)  [unwired: 8 in, 1 out]
